vi "Query with 1D String Result.vi"(8 "error in (no error)":errorcluster, 10 "Query string":string, 11 "IDatabase in":refnum<class "IDatabase.lvclass">) -> (0 "error out":errorcluster, 2 "Result":string[](array[string]), 3 "IDatabase out":refnum<class "IDatabase.lvclass">)   [LabVIEW 2020, in "IDatabase.lvlib" / "IDatabase.lvclass"]
uses:
  IDatabase.lvclass
  <vilib>/Utility/error.llb/Error Cluster From Error Code.vi
  <vilib>/ErrorRing/Error Ring.xnode
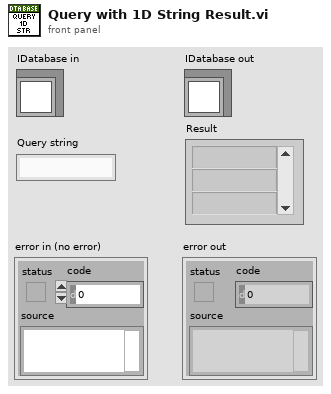
[diagram p1: front panel]
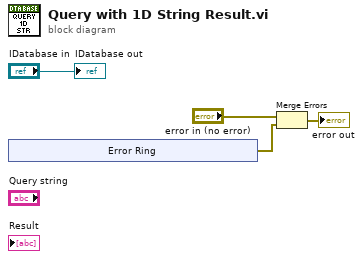
[diagram p0: block diagram]
diagram:
  n1 = xnode "Error Ring"() -> ("error out"=w3:errorcluster)
  n2 = Merge Errors("error in (no error)", w3) -> (→"error out":errorcluster)
  "IDatabase out" <- "IDatabase in"
